vi "Camera.vi"   [LabVIEW 2015]
panel:
  # "By: Joshua Merkle 1/25/16"
types:
  T1 = typedef "WPI_CameraDevRef.ctl" = cluster{"Camera Address":string, "CameraStatus":errorcluster}
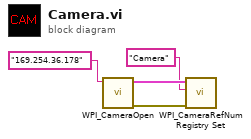
[diagram p0: block diagram]
diagram:
  n1 = call <vilib>:"WPI_CameraOpen.vi"("Camera Address"="169.254.36.178") -> ("error out"=w4:errorcluster, "CameraDevRef"=w3:T1)  [unwired: 9 in]
  n2 = call <vilib>:"WPI_CameraRefNum Registry Set.vi"("error in (no error)"=w4, "refnum name"="Camera", "CameraDevRef"=w3) -> ()  [unwired: 7 in, 2 out]
